vi "Front Panel.vi"() -> ()   [LabVIEW 2021]
panel:
  out "Puzzle Bounds":T1
  in  "buffer":u32
  in  "Clear":bool
  out "Puzzle":picture
  in  "Exit":bool
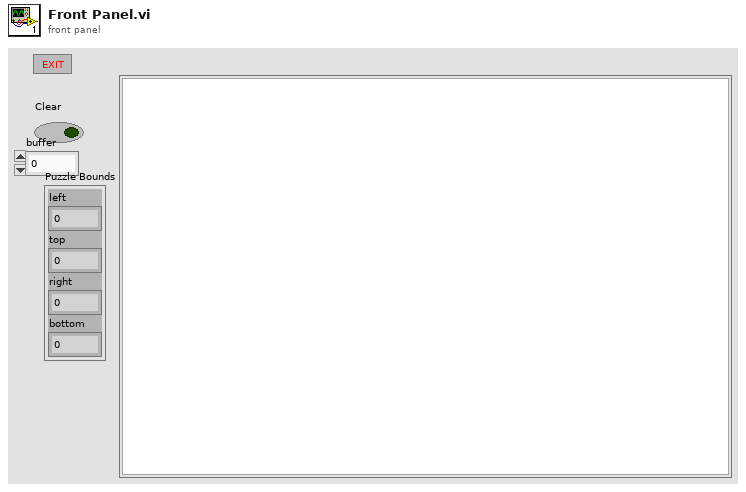
[diagram p1: front panel]
types:
  T1 = cluster{"left":i16, "top":i16, "right":i16, "bottom":i16}
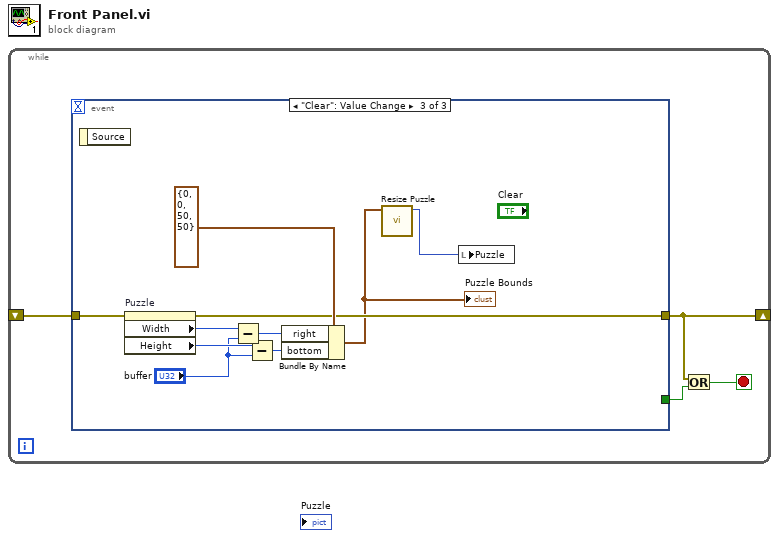
[diagram p0: block diagram]
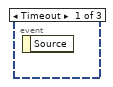
[diagram p2: hidden frame]
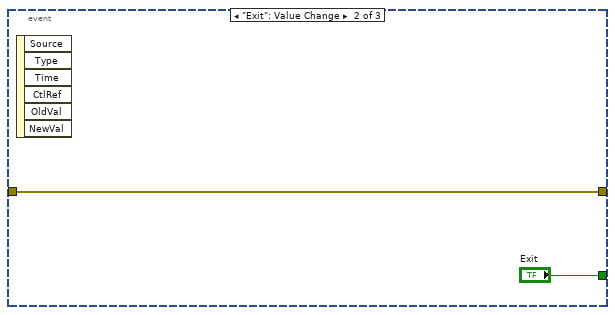
[diagram p3: hidden frame]
diagram:
  n1 = while {
    shift-right: [w1] -> _
    shift-left: _ -> [w4]
    stop <- w2 stop-if-true
    n2 = event shown="[2] \"Clear\": Value Change" {
      selector: _ -> [_ _ _]
      dyn-events: _ -> [_ _ _]
      timeout: _ -> [_ _ _]
      tunnel: [_ "Exit" _] -> w3
      tunnel: [_ w5 w14] -> w1
      tunnel: w4 -> [_ w5 w15]
      event Timeout {
        n3 = event-data() -> ()  [unwired: 1 in, 1 out]
      }
      event "Exit": Value Change {
        n4 = event-data() -> ()  [unwired: 1 in, 6 out]
      }
      event "Clear": Value Change {
        n5 = event-data() -> ()  [unwired: 1 in, 1 out]
        n6 = property on="Puzzle" class="Pict"(error in=w15) -> (error out=w14:errorcluster, "Width"=w13:u32, "Height"=w11:u32)  [unwired: 1 in, 1 out]
        n7 = Subtract(x=w13, y="buffer") -> (x-y=w12:u32)
        n8 = Subtract(x=w11, y="buffer") -> (x-y=w9:u32)
        n9 = Bundle By Name(cluster=T1 {"left"=0, "top"=0, "right"=50, "bottom"=50} ("rect"), "right"=w12, "bottom"=w9) -> (w7:T1)
        "Puzzle Bounds" <- w7
        n10 = call "Resize Puzzle.vi"("Puzzle Bounds"=w7) -> ("picture"=w8:picture)  [unwired: 10 in]
        n11 = local write "Puzzle"(w8) -> ()
      }
    }
    n12 = Or(x=w1, y=w3) -> (x .or. y?=w2:bool)
  }
